vi "Colour Image to Numpy Array.vi"(8 "error in (no error)":errorcluster, 11 "Refnum in":T1) -> (0 "error out":errorcluster, 3 "Array":u8[][][](array[numeric]))   [LabVIEW 2022 SP3]
doc: "OpenCV can take an image as a 3d numpy array.\n\nThis converts a colour image to that format - with 3 dimensions for each colour plane."
uses:
  <vilib>/vision/Image Controls.llb/IMAQ Image.ctl
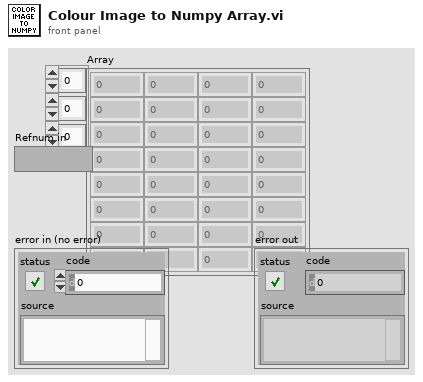
[diagram p1: front panel]
types:
  T1 = typedef "IMAQ Image.ctl" = refnum<image>
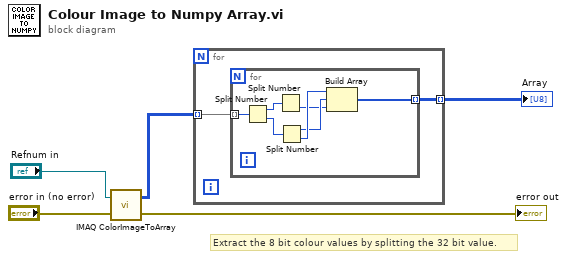
[diagram p0: block diagram]
diagram:
  # "Extract the 8 bit colour values by splitting the 32 bit value."
  n1 = call "IMAQ ColorImageToArray"("Image"="Refnum in", "error in (no error)"="error in (no error)") -> ("Image Pixels (U32)"=w2:u32[][], "error out"=→"error out":errorcluster)  [unwired: 2 in, 1 out]
  n2 = for {
    tunnel: w2 -> [w7] mode=indexing
    tunnel: [w6] -> w1 mode=indexing
    n3 = for {
      tunnel: w7 -> [w14] mode=indexing
      tunnel: [w11] -> w6 mode=indexing
      n4 = Split Number(x=w14) -> (hi(x)=w13:u16, lo(x)=w12:u16)
      n5 = Split Number(x=w13) -> (lo(x)=w8:u8)  [unwired: 1 out]
      n6 = Split Number(x=w12) -> (hi(x)=w9:u8, lo(x)=w10:u8)
      n7 = Build Array(w10, w9, w8) -> (w11:u8[])
    }
  }
  "Array" <- w1
